vi "FindTargetIndex.vi"(11 "Selected Target":i32) -> (3 "Target Index":i32)   [LabVIEW 2011]
uses:
  Robot Global Data.vi
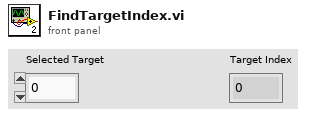
[diagram p1: front panel]
types:
  T1 = cluster{"Position":cluster{"X":dbl, "Y":dbl}, "Distance (ft)":dbl}[]
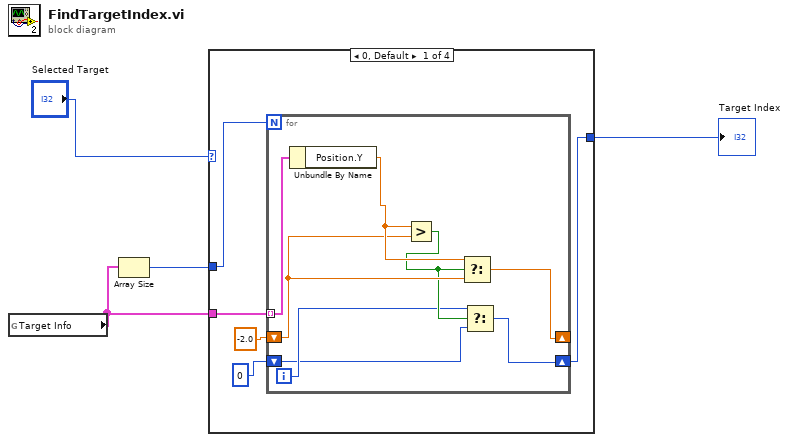
[diagram p0: block diagram]
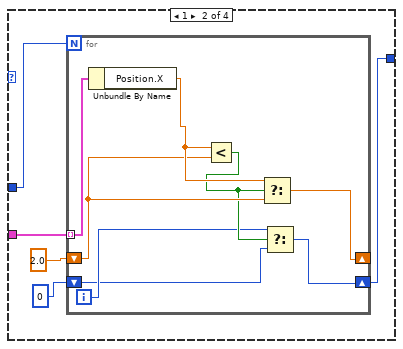
[diagram p2: hidden frame]
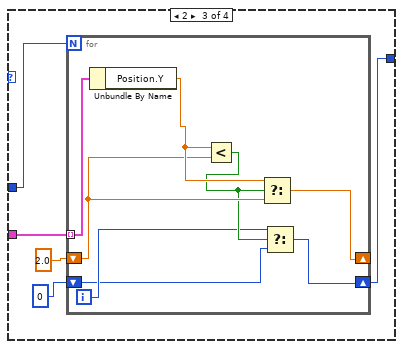
[diagram p3: hidden frame]
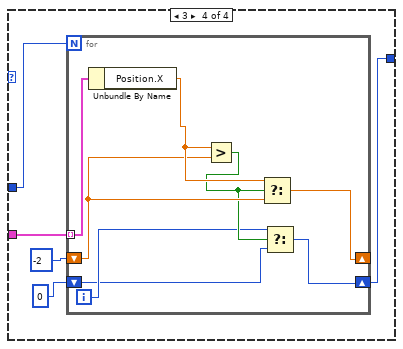
[diagram p4: hidden frame]
diagram:
  n1 = global read "Robot Global Data.vi" "Target Info"() -> (w2:T1)
  n2 = Array Size(array=w2) -> (size(s)=w3:i32)
  n3 = case shown="0, Default" "Selected Target" {
    tunnel: w3 -> [w9 w22 w35 w48]
    tunnel: w2 -> [w8 w21 w34 w47]
    tunnel: [w5 w18 w31 w44] -> w1
    frame 0, Default {
      n4 = for {
        N: w9 -> [_]
        shift-right: [w14] -> _
        shift-left: -2.0 -> [w15]
        tunnel: w8 -> [w17] mode=indexing
        shift-right: [w10] -> w5
        shift-left: 0 -> [w11]
        i -> [w12]
        n5 = Unbundle By Name(w17) -> ("Position.Y"=w16:dbl)
        n6 = Greater?(x=w16, y=w15) -> (0:w13:bool)
        n7 = Select(t=w16, s=w13, f=w15) -> (s? t:f=w14:dbl)
        n8 = Select(t=w12, s=w13, f=w11) -> (s? t:f=w10:i32)
      }
    }
    frame 1 {
      n9 = for {
        N: w22 -> [_]
        shift-right: [w27] -> _
        shift-left: 2.0 -> [w28]
        tunnel: w21 -> [w30] mode=indexing
        shift-right: [w23] -> w18
        shift-left: 0 -> [w24]
        i -> [w25]
        n10 = Unbundle By Name(w30) -> ("Position.X"=w29:dbl)
        n11 = Less?(x=w29, y=w28) -> (x < y?=w26:bool)
        n12 = Select(t=w29, s=w26, f=w28) -> (s? t:f=w27:dbl)
        n13 = Select(t=w25, s=w26, f=w24) -> (s? t:f=w23:i32)
      }
    }
    frame 2 {
      n14 = for {
        N: w35 -> [_]
        shift-right: [w40] -> _
        shift-left: 2.0 -> [w41]
        tunnel: w34 -> [w43] mode=indexing
        shift-right: [w36] -> w31
        shift-left: 0 -> [w37]
        i -> [w38]
        n15 = Unbundle By Name(w43) -> ("Position.Y"=w42:dbl)
        n16 = Less?(x=w42, y=w41) -> (x < y?=w39:bool)
        n17 = Select(t=w42, s=w39, f=w41) -> (s? t:f=w40:dbl)
        n18 = Select(t=w38, s=w39, f=w37) -> (s? t:f=w36:i32)
      }
    }
    frame 3 {
      n19 = for {
        N: w48 -> [_]
        shift-right: [w53] -> _
        shift-left: -2 -> [w54]
        tunnel: w47 -> [w56] mode=indexing
        shift-right: [w49] -> w44
        shift-left: 0 -> [w50]
        i -> [w51]
        n20 = Unbundle By Name(w56) -> ("Position.X"=w55:dbl)
        n21 = Greater?(x=w55, y=w54) -> (0:w52:bool)
        n22 = Select(t=w55, s=w52, f=w54) -> (s? t:f=w53:dbl)
        n23 = Select(t=w51, s=w52, f=w50) -> (s? t:f=w49:i32)
      }
    }
  }
  "Target Index" <- w1
